vi "Create Cursor Z Data.vi"(8 "error in":errorcluster, 10 "Images":refnum<queue>, 11 "Graph with Series View in":refnum<class "Graph with Series View.lvclass">) -> (0 "error out":errorcluster, 2 "Cursor Z U16":u16[](array[numeric]), 3 "Graph with Series View out":refnum<class "Graph with Series View.lvclass">)   [LabVIEW 2025, in "Graph with Series View.lvclass"]
uses:
  Graph with Series View.lvclass
  HAL/Source/Typedefs/Generic Image/Generic Image.lvclass
  Base Graph/Base Graph.lvclass/Base Graph.ctl
  Base Graph/Base Graph.lvclass
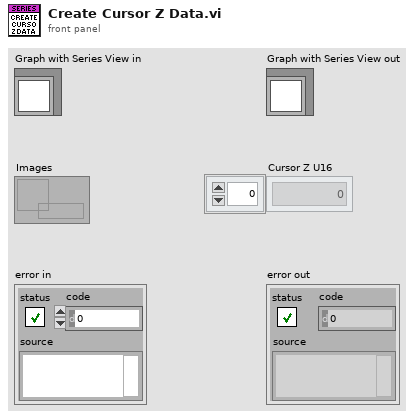
[diagram p1: front panel]
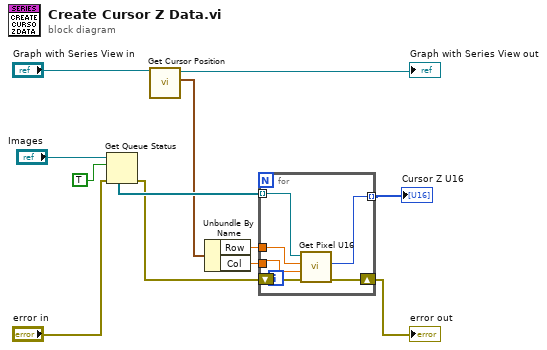
[diagram p0: block diagram]
diagram:
  n1 = Get Queue Status(queue="Images", return elements? (F)=TRUE, error in (no error)="error in") -> (error out=w1:errorcluster, elements=w10:refnum<class "Generic Image.lvclass">[])  [unwired: 6 out]
  n2 = call "Get Cursor Position.vi"("Base Graph in"="Graph with Series View in") -> ("Cursor Position"=w6:cluster{"Col":dbl, "Row":dbl}, "Base Graph out"=→"Graph with Series View out":refnum<class "Graph with Series View.lvclass">)  [unwired: 9 in]
  n3 = Unbundle By Name(w6) -> ("Row"=w5:dbl, "Col"=w4:dbl)
  n4 = for {
    tunnel: w10 -> [w18] mode=indexing
    tunnel: w5 -> [w14]
    tunnel: w4 -> [w13]
    shift-right: [w16] -> w9
    shift-left: w1 -> [w17]
    tunnel: [w15] -> w3 mode=indexing
    n5 = call-dynamic "Get Pixel U16.vi"("error in"=w17, "col"=w13, "row"=w14, "Generic Image in"=w18) -> ("error out"=w16:errorcluster, "Pixel"=w15:u16)  [unwired: 6 in]
  }
  "error out" <- w9
  "Cursor Z U16" <- w3
